vi "Pipelining.vi"() -> ()   [LabVIEW 2012]
uses:
  <vilib>/Platform/TimedLoop/XDataNode/timing_clust.ctl
  <vilib>/Platform/TimedLoop/XDataNode/nitl_modes.ctl
  <vilib>/Platform/TimedLoop/XDataNode/wakeup.ctl
  <vilib>/rvi/Emulation/niFpgaSctlEmulationRegisterWithScheduler.vi
  <vilib>/rvi/Emulation/niFpgaSctlEmulationScheduler.vi
  <vilib>/Platform/TimedLoop/XDataNode/XDataNode.xnode
  <vilib>/Platform/TimedLoop/XDataNode/XDNodeRunTimeDep.lvlib
panel:
  out "Result":u32
  in  "Input":u32=1000
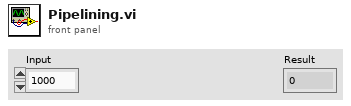
[diagram p1: front panel]
types:
  T1 = typedef "XDNodeRunTimeDep.lvlib/timing_clust.ctl" = cluster{"Expected End [f-1]":u64, "Actual End [f-1]":u64, "Finished Late? [f-1]":bool, "Expected End [i-1]":u64, "Actual End [i-1]":u64, "Finished Late? [i-1]":bool, "Expected Start [i]":u64, "Actual Start [i]":u64, "Expected Start [f]":u64, "Actual Start [f]":u64, "Source Name":string, "Structure Name":string, "Period":i64, "Deadline":i64, "Offset":i64, "Start":i64, "Priority":i32, "Timeout":i32, "Mode":T2, "Wakeup Reason":T3, "Error":errorcluster, "Source Type":string, "Secondary Source Type":string, "Global End Time":u64, "Global Start Time":u64, "Frame Duration":u64, "Iteration Duration":u64, "Assigned CPU":i32, "I/O Scan Engine Mode":u32}
  T2 = typedef "XDNodeRunTimeDep.lvlib/nitl_modes.ctl" = enum32{"No Change", "Process missed periods, maintain original phase", "Discard missed periods, maintain original phase", "Process missed periods, ignore original phase", "Discard missed periods, ignore original phase"}
  T3 = typedef "XDNodeRunTimeDep.lvlib/wakeup.ctl" = enum32{"Normal", "Aborted", "Asynchronous wakeup", "Timing source error", "Timed loop error", "Timeout"}
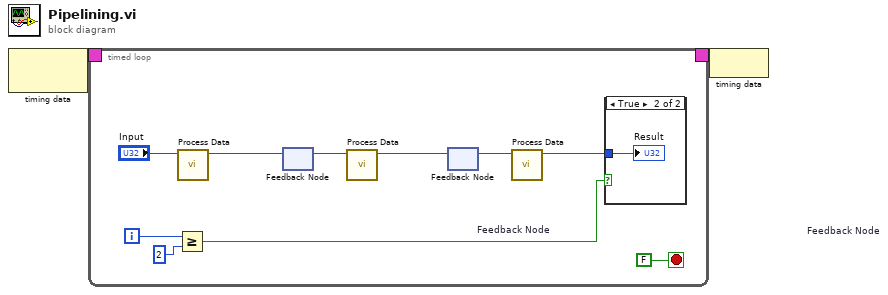
[diagram p0: block diagram]
diagram:
  n1 = node-c288() -> (w2:T1)  [unwired: 1 in]
  n2 = timed-loop {
    timing: w2 -> [_]
    timing-out: [_] -> w1
    i -> [w5]
    stop <- FALSE stop-if-true
    n3 = Greater Or Equal?(x=w5, y=2) -> (x >= y?=w3:bool)
    n4 = call "Process Data.vi"("x"="Input") -> ("Result"=w10:u32)  [unwired: 10 in]
    n5 = feedback-in #1(w10) -> ()
    n6 = feedback #1 "Feedback Node"() -> (w9:u32)  [unwired: 1 in]
    n7 = call "Process Data.vi"("x"=w9) -> ("Result"=w8:u32)  [unwired: 10 in]
    n8 = feedback #2 "Feedback Node"() -> (w7:u32)  [unwired: 1 in]
    n9 = feedback-in #2(w8) -> ()
    n10 = call "Process Data.vi"("x"=w7) -> ("Result"=w6:u32)  [unwired: 10 in]
    n11 = case shown="True" w3 {
      tunnel: w6 -> [_ w13]
      frame False {
      }
      frame True {
        "Result" <- w13
      }
    }
  }
  n12 = node-c288(w1) -> ()
